vi "Timestamp to ISO-8601 UTC.vi"(7 "Now for Unset? (T)":bool=TRUE, 11 "Time Stamp":timestamp) -> (3 "ISO 8601 UTC":string)   [LabVIEW 2018, in "JSON.lvlib"]
uses:
  JSON.lvlib
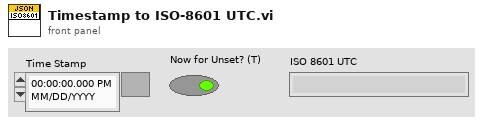
[diagram p1: front panel]
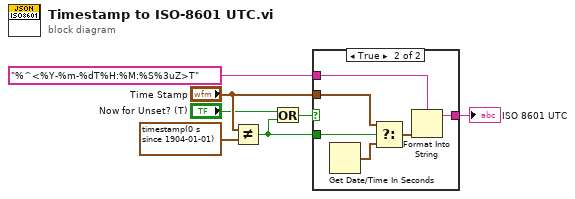
[diagram p0: block diagram]
diagram:
  n1 = Not Equal?(x="Time Stamp", y=timestamp(0 s since 1904-01-01)) -> (x != y?=w2:bool)
  n2 = Or(x="Now for Unset? (T)", y=w2) -> (x .or. y?=w1:bool)
  n3 = case shown="True" w1 {
    tunnel: "%^<%Y-%m-%dT%H:%M:%S%3uZ>T" ("format string") -> [_ w13]
    tunnel: [_ w12] -> w6
    tunnel: "Time Stamp" -> [_ w11]
    tunnel: w2 -> [_ w9]
    frame False {
    }
    frame True {
      n4 = Get Date/Time In Seconds() -> (seconds since 1Jan1904=w10:timestamp)
      n5 = Select(t=w11, s=w9, f=w10) -> (s? t:f=w8:timestamp)
      n6 = Format Into String(format string=w13, w8) -> (resulting string=w12:string)  [unwired: 2 in, 1 out]
    }
  }
  "ISO 8601 UTC" <- w6
